vi "Hex String To Ascll.vi"(10 "HEX String":string) -> (2 "Ascll":string)   [LabVIEW 2017]
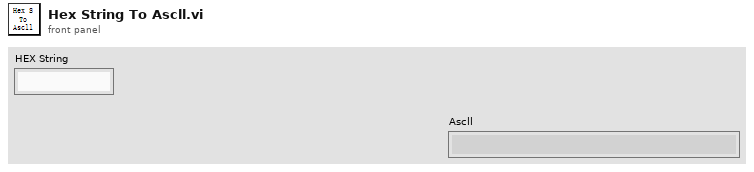
[diagram p1: front panel]
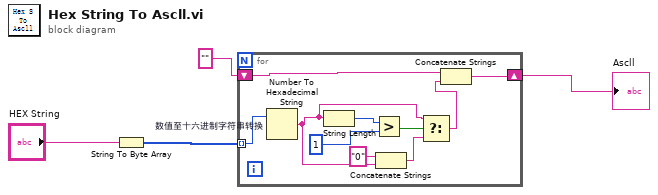
[diagram p0: block diagram]
diagram:
  n1 = String To Byte Array ("字符串至字节数组转换")(string="HEX String") -> (unsigned byte array=w1:u8[])
  n2 = for {
    tunnel: w1 -> [w14] mode=indexing
    shift-right: [w12] -> w2
    shift-left: "" -> [w13]
    n3 = Number To Hexadecimal String "数值至十六进制字符串转换"(2:w14) -> (0:w6:string)  [unwired: 1 in]
    n4 = String Length(string=w6) -> (length=w11:i32)
    n5 = Greater?(x=w11, y=1) -> (0:w9:bool)
    n6 = Concatenate Strings("0" ("字符串"), w6) -> (w7:string)
    n7 = Select(t=w6, s=w9, f=w7) -> (s? t:f=w8:string)
    n8 = Concatenate Strings(w13, w8) -> (w12:string)
  }
  "Ascll" <- w2
